vi "OpenClose.vi"(5 "FastOpen?":bool, 7 "Open/Close":T1=enum."Open", 8 "error in":errorcluster, 11 "References":T2) -> (0 "error out":errorcluster)   [LabVIEW 2021]
uses:
  Typedefs/Referencias.ctl
  Typedefs/Axis.ctl
  Typedefs/OpenClose.ctl
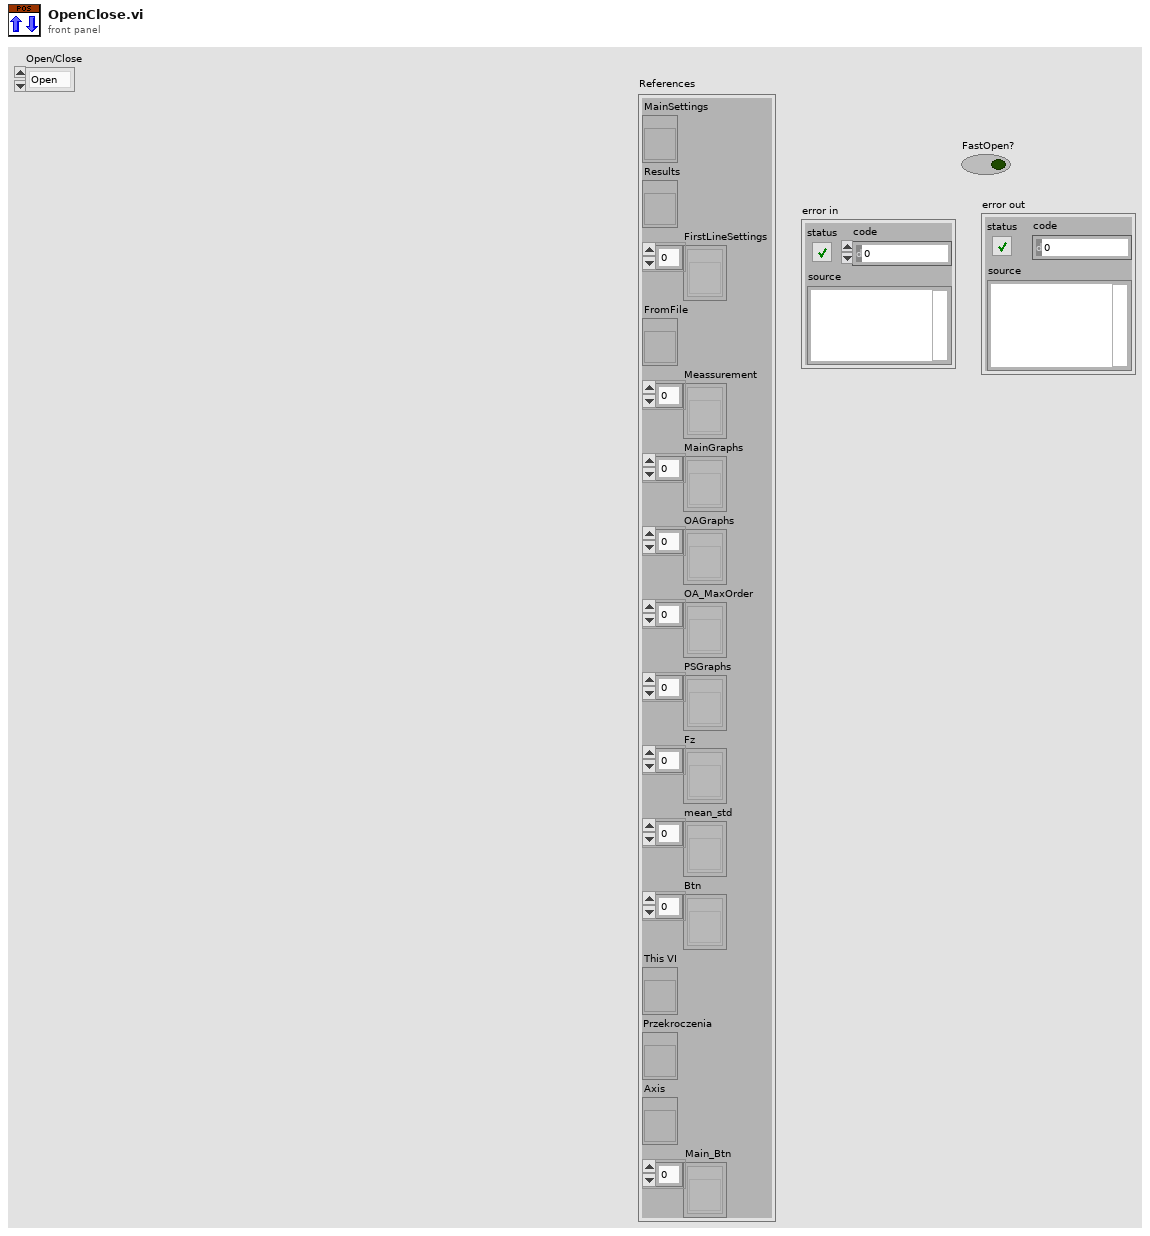
[diagram p1: front panel]
types:
  T1 = typedef "OpenClose.ctl" = enum16{"Close", "Open"}
  T2 = typedef "Referencias.ctl" = cluster{"MainSettings":refnum<vi>, "Results":refnum<vi>, "FirstLineSettings":refnum<vi>[], "FromFile":refnum<vi>, "Meassurement":refnum<vi>[], "MainGraphs":refnum<vi>[], "OAGraphs":refnum<vi>[], "OA_MaxOrder":refnum<vi>[], "PSGraphs":refnum<vi>[], "Fz":refnum<vi>[], "mean_std":refnum<vi>[], "Btn":refnum<vi>[], "This VI":refnum<vi>, "Przekroczenia":refnum<vi>, "Axis":refnum<vi>, "Main_Btn":refnum<vi>[]}
  T3 = typedef "LVPointTypeDef.ctl" = cluster{"Horizontal":i16, "Vertical":i16}
  T4 = typedef "LVPositionTypeDef.ctl" = cluster{"Left":i32, "Top":i32}
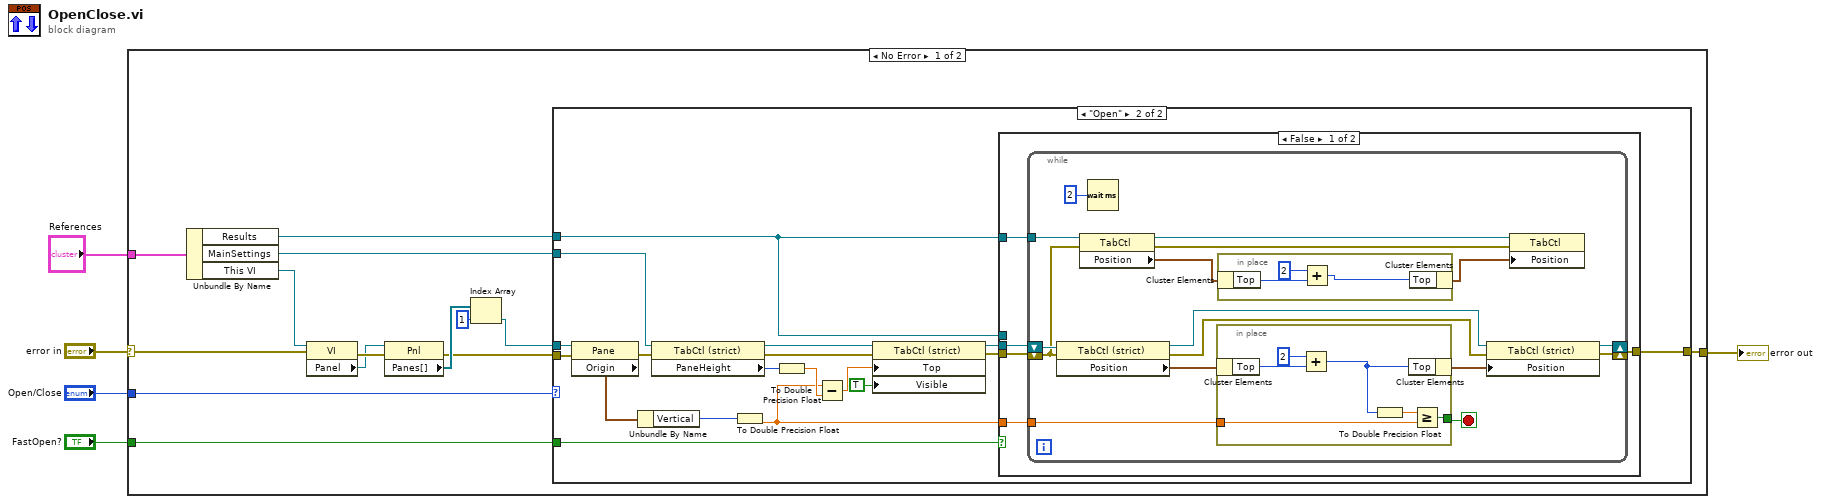
[diagram p0: block diagram]
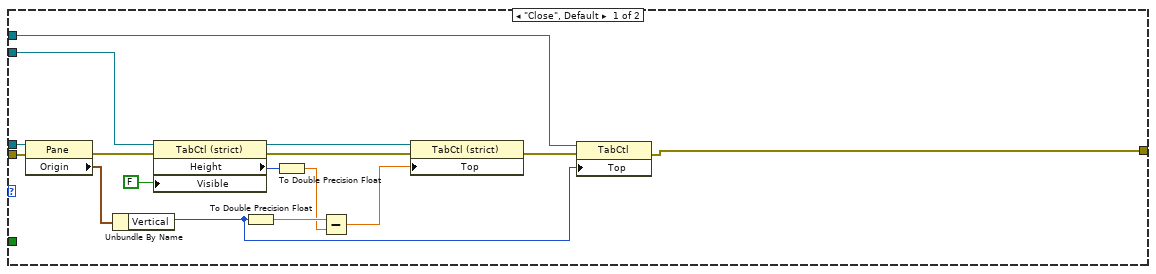
[diagram p2: hidden frame]
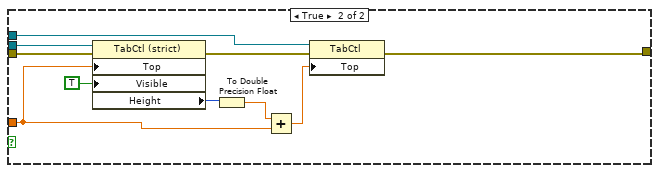
[diagram p3: hidden frame]
diagram:
  n1 = case shown="No Error" "error in" {
    selector: "error in" -> [w7 w94]
    tunnel: [w19 w94] -> w5
    tunnel: "Open/Close" -> [w18 _]
    tunnel: "References" -> [w17 _]
    tunnel: "FastOpen?" -> [w16 _]
    frame No Error {
      n2 = Unbundle By Name(w17) -> ("Results"=w6:refnum<vi>, "MainSettings"=w15:refnum<vi>, "This VI"=w8:refnum<vi>)
      n3 = property class="VI"(reference=w8, error in=w7) -> (error out=w14:errorcluster, "Panel"=w13:refnum<vi>)  [unwired: 1 out]
      n4 = property class="Pnl"(reference=w13, error in=w14) -> (error out=w10:errorcluster, "Panes[]"=w12:refnum<vi>[])  [unwired: 1 out]
      n5 = Index Array(array=w12, index=1) -> (element=w9:refnum<vi>)
      n6 = case shown="\"Open\"" w18 {
        tunnel: [w20 w51] -> w19
        tunnel: w9 -> [w30 w50]
        tunnel: w10 -> [w29 w49]
        tunnel: w16 -> [_ w45]
        tunnel: w15 -> [w28 w42]
        tunnel: w6 -> [w22 w36]
        frame "Close", Default {
          n7 = property class="Pane"(reference=w30, error in=w29) -> (error out=w34:errorcluster, "Origin"=w24:T3)  [unwired: 1 out]
          n8 = Unbundle By Name(w24) -> ("Vertical"=w21:i16)
          n9 = property class="TabCtl (strict)"(reference=w28, error in=w34, "Visible"=FALSE) -> (reference out=w32:refnum<vi>, error out=w33:errorcluster, "Height"=w26:u32)
          n10 = To Double Precision Float(number=w21) -> (double precision float=w27:dbl)
          n11 = To Double Precision Float(number=w26) -> (double precision float=w25:dbl)
          n12 = Subtract(x=w27, y=w25) -> (x-y=w31:dbl)
          n13 = property class="TabCtl (strict)"(reference=w32, error in=w33, "Top"=w31) -> (error out=w23:errorcluster)  [unwired: 1 out]
          n14 = property class="TabCtl"(reference=w22, error in=w23, "Top"=w21) -> (error out=w20:errorcluster)  [unwired: 1 out]
        }
        frame "Open" {
          n15 = property class="Pane"(reference=w50, error in=w49) -> (error out=w48:errorcluster, "Origin"=w38:T3)  [unwired: 1 out]
          n16 = Unbundle By Name(w38) -> ("Vertical"=w37:i16)
          n17 = property class="TabCtl (strict)"(reference=w42, error in=w48) -> (reference out=w46:refnum<vi>, error out=w47:errorcluster, "PaneHeight"=w41:u32)
          n18 = To Double Precision Float(number=w37) -> (double precision float=w39:dbl)
          n19 = To Double Precision Float(number=w41) -> (double precision float=w40:dbl)
          n20 = Subtract(x=w39, y=w40) -> (x-y=w44:dbl)
          n21 = property class="TabCtl (strict)"(reference=w46, error in=w47, "Top"=w44, "Visible"=TRUE) -> (reference out=w52:refnum<vi>, error out=w53:errorcluster)
          n22 = case shown="False" w45 {
            tunnel: w53 -> [w58 w93]
            tunnel: w52 -> [w57 w92]
            tunnel: [w56 w89] -> w51
            tunnel: w39 -> [w55 w85]
            tunnel: w36 -> [_ w88]
            tunnel: w36 -> [w54 _]
            frame False {
              n23 = while {
                shift-right: [w70] -> w56
                shift-left: w58 -> [w61]
                tunnel: w55 -> [w68]
                shift-right: [w65] -> _
                shift-left: w57 -> [w66]
                tunnel: w54 -> [w62]
                stop <- w67 stop-if-true
                n24 = property on="Property Node" class="TabCtl (strict)"(reference=w66, error in=w61) -> (reference out=w69:refnum<vi>, error out=w71:errorcluster, "Position"=w74:T4)
                n25 = property on="Property Node" class="TabCtl"(reference=w62, error in=w61) -> (reference out=w63:refnum<vi>, error out=w64:errorcluster, "Position"=w60:T4)
                n26 = Wait (ms)(milliseconds to wait=u32 2) -> ()  [unwired: 1 out]
                n27 = in-place {
                  in-place-border: w68 -> [w82]
                  in-place-border: [w83] -> w67
                  n28 = in-place-cluster #1(w74) -> ("Top"=w80:i32)
                  n29 = Add(x=2, y=w80) -> (x+y=w79:i32)
                  n30 = To Double Precision Float(number=w79) -> (double precision float=w81:dbl)
                  n31 = in-place-cluster #1("Top"=w79) -> (w73:T4)
                  n32 = Greater Or Equal?(x=w81, y=w82) -> (x >= y?=w83:bool)
                }
                n33 = in-place {
                  n34 = in-place-cluster #2(w60) -> ("Top"=w77:i32)
                  n35 = Add(x=2, y=w77) -> (x+y=w76:i32)
                  n36 = in-place-cluster #2("Top"=w76) -> (w59:T4)
                }
                n37 = property on="Property Node" class="TabCtl (strict)"(reference=w69, error in=w71, "Position"=w73) -> (reference out=w65:refnum<vi>, error out=w70:errorcluster)
                n38 = property on="Property Node" class="TabCtl"(reference=w63, error in=w64, "Position"=w59) -> ()  [unwired: 2 out]
              }
            }
            frame True {
              n39 = property on="Property Node" class="TabCtl (strict)"(reference=w92, error in=w93, "Top"=w85, "Visible"=TRUE) -> (error out=w90:errorcluster, "Height"=w87:u32)  [unwired: 1 out]
              n40 = To Double Precision Float(number=w87) -> (double precision float=w86:dbl)
              n41 = Add(x=w86, y=w85) -> (x+y=w84:dbl)
              n42 = property on="Property Node" class="TabCtl"(reference=w88, error in=w90, "Top"=w84) -> (error out=w89:errorcluster)  [unwired: 1 out]
            }
          }
        }
      }
    }
    frame Error {
    }
  }
  "error out" <- w5
